vi "Dashboard Resize.vi"(6 "Cluster":T2={"Label Font Size"=24, "Data Font Size"=36, "String Font Size"=36}, 7 "Cluster 2":T1={"Label(%)"=0.4, "Data(%)"=0.4, "String(%)"=0.2}, 8 "error in (no error)":errorcluster, 9 "Cluster Size:Height":u32=134, 10 "Cluster Size:Width":u32=256, 11 "ClusterRef":refnum<vi>) -> (0 "error out":errorcluster, 1 "Bounds:Area Height":u32=134, 2 "Bounds:Area Width":u32=256)   [LabVIEW 2020, in "CSM-TagDashboard.lvlib"]
doc: "-- <b>Controls</b> --\n- <b>Cluster</b>:\n- <b>Cluster Size:Height</b>:\n- <b>Cluster Size:Width</b>:\n- <b>ClusterRef</b>:\n\n-- <b>Indicators</b> --\n- <b>Bounds:Area Height</b>:\n- <b>Bounds:Area Width</b>:"
uses:
  CSM-TagDashboard.lvlib
panel:
  out "引气压力P4 2":T3={"Label"="Label", "Value"="0.00", "String"="0.00"} caption="Digital"
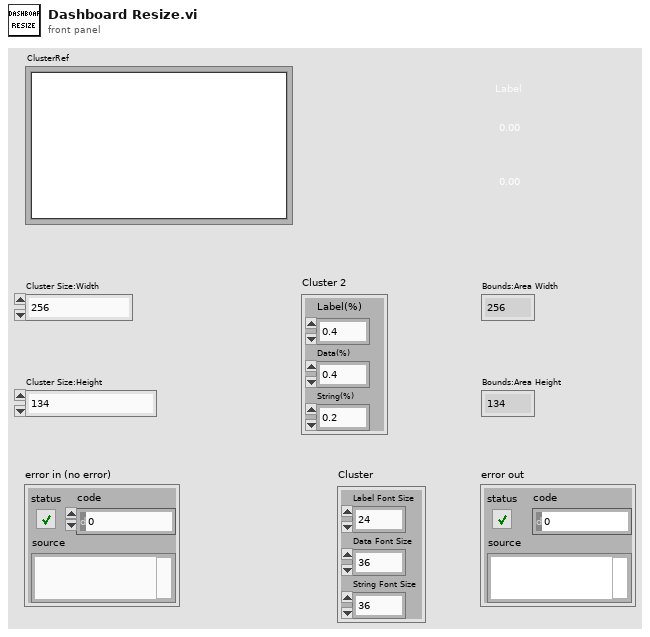
[diagram p1: front panel]
types:
  T1 = cluster{"Label(%)":dbl, "Data(%)":dbl, "String(%)":dbl}
  T2 = cluster{"Label Font Size":i32, "Data Font Size":i32, "String Font Size":i32}
  T3 = cluster{"Label":string, "Value":string, "String":string}
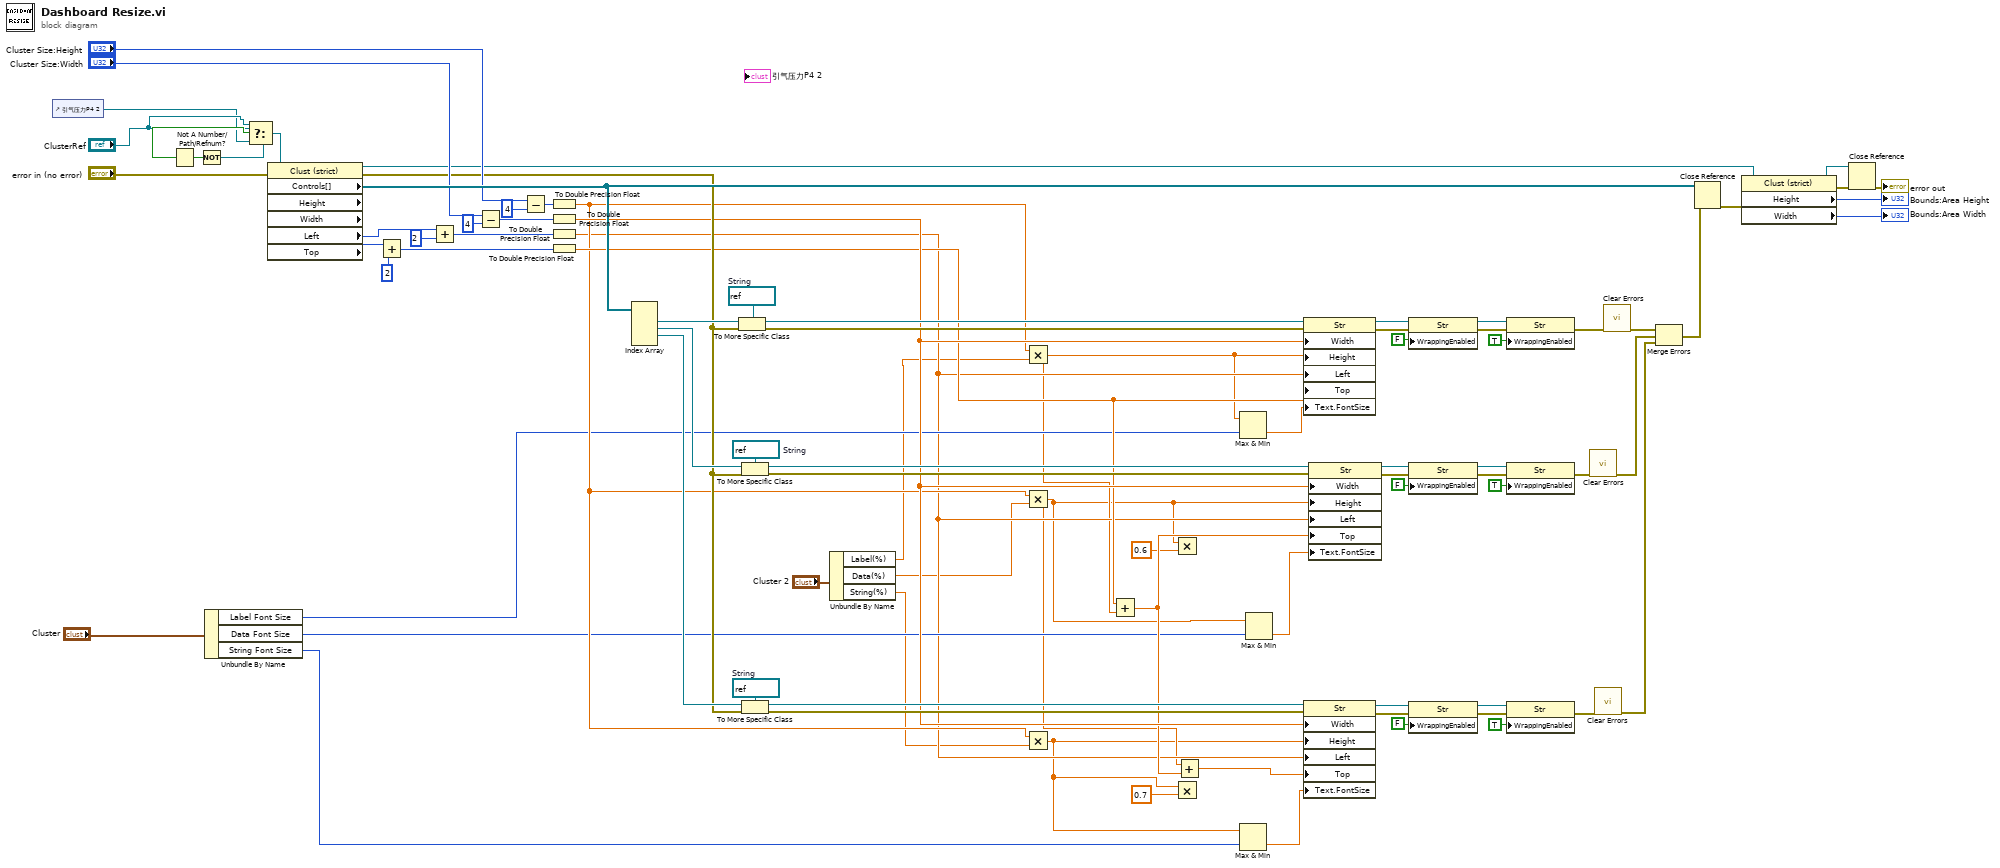
[diagram p0: block diagram]
diagram:
  w50 = refnum<vi> refnum  # String
  w81 = refnum<vi> refnum  # String
  w85 = refnum<vi> refnum  # String
  n1 = control-ref of="引气压力P4 2"() -> (w56:refnum<vi>)
  n2 = Not A Number/Path/Refnum?(number/path/refnum="ClusterRef") -> (NaN/Path/Refnum?=w15:bool)
  n3 = Not(x=w15) -> (.not. x?=w58:bool)
  n4 = Unbundle By Name("Cluster") -> ("Label Font Size"=w14:i32, "Data Font Size"=w13:i32, "String Font Size"=w12:i32)
  n5 = Select(t="ClusterRef", s=w58, f=w56) -> (s? t:f=w55:refnum<vi>)
  n6 = property on="Property Node" class="Clust (strict)" props=["Controls[]", "Height", "Width", "Left", "Top"](reference=w55, error in="error in (no error)") -> (reference out=w62:refnum<vi>, error out=w47:errorcluster, "Controls[]"=w86:refnum<vi>[], "Left"=w75:i32, "Top"=w72:i32)  [unwired: 2 out]
  n7 = Add(x=w72, y=2) -> (x+y=w53:i32)
  n8 = Add(x=w75, y=2) -> (x+y=w71:i32)
  n9 = Subtract(x="Cluster Size:Width", y=u32 4) -> (x-y=w78:u32)
  n10 = Subtract(x="Cluster Size:Height", y=u32 4) -> (x-y=w54:u32)
  n11 = To Double Precision Float(number=w54) -> (double precision float=w40:dbl)
  n12 = To Double Precision Float(number=w78) -> (double precision float=w46:dbl)
  n13 = To Double Precision Float(number=w71) -> (double precision float=w11:dbl)
  n14 = To Double Precision Float(number=w53) -> (double precision float=w42:dbl)
  n15 = Index Array(array=w86) -> (element #1=w83:refnum<vi>, element #2=w80:refnum<vi>, element #3=w48:refnum<vi>)  [unwired: 4 in, 1 out]
  n16 = To More Specific Class(target class=w85, reference=w83, error in=w47) -> (specific class reference=w84:refnum<vi>, error out=w68:errorcluster)
  n17 = To More Specific Class(target class=w81, reference=w80, error in=w47) -> (specific class reference=w82:refnum<vi>, error out=w69:errorcluster)
  n18 = To More Specific Class(target class=w50, reference=w48, error in=w47) -> (specific class reference=w49:refnum<vi>, error out=w51:errorcluster)
  n19 = Unbundle By Name("Cluster 2") -> ("Label(%)"=w7:dbl, "Data(%)"=w8:dbl, "String(%)"=w9:dbl)
  n20 = Multiply(x=w40, y=w7) -> (x*y=w3:dbl)
  n21 = Multiply(x=w40, y=w8) -> (x*y=w2:dbl)
  n22 = Multiply(x=w40, y=w9) -> (x*y=w1:dbl)
  n23 = Add(x=w42, y=w3) -> (x+y=w45:dbl)
  n24 = Multiply(x=w2, y=0.6) -> ()  [unwired: 1 out]
  n25 = Multiply(x=w1, y=0.7) -> ()  [unwired: 1 out]
  n26 = Add(x=w2, y=w45) -> (x+y=w52:dbl)
  n27 = Max & Min(x=w3, y=w14) -> (min(x,y)=w6:dbl)  [unwired: 1 out]
  n28 = Max & Min(x=w1, y=w12) -> (min(x,y)=w4:dbl)  [unwired: 1 out]
  n29 = Max & Min(x=w2, y=w13) -> (min(x,y)=w5:dbl)  [unwired: 1 out]
  n30 = property on="Property Node" class="Str"(reference=w84, error in=w68, "Width"=w46, "Height"=w3, "Left"=w11, "Top"=w42, "Text.FontSize"=w6) -> (reference out=w36:refnum<vi>, error out=w35:errorcluster)
  n31 = property on="Property Node" class="Str"(reference=w49, error in=w51, "Width"=w46, "Height"=w1, "Left"=w11, "Top"=w52, "Text.FontSize"=w4) -> (reference out=w18:refnum<vi>, error out=w17:errorcluster)
  n32 = property on="Property Node" class="Str"(reference=w82, error in=w69, "Width"=w46, "Height"=w2, "Left"=w11, "Top"=w45, "Text.FontSize"=w5) -> (reference out=w24:refnum<vi>, error out=w25:errorcluster)
  n33 = property on="Property Node" class="Str"(reference=w36, error in=w35, "WrappingEnabled"=FALSE ("Enable Wrapping")) -> (reference out=w31:refnum<vi>, error out=w32:errorcluster)
  n34 = property on="Property Node" class="Str"(reference=w24, error in=w25, "WrappingEnabled"=FALSE ("Enable Wrapping")) -> (reference out=w29:refnum<vi>, error out=w28:errorcluster)
  n35 = property on="Property Node" class="Str"(reference=w18, error in=w17, "WrappingEnabled"=FALSE ("Enable Wrapping")) -> (reference out=w19:refnum<vi>, error out=w20:errorcluster)
  n36 = property on="Property Node" class="Str"(reference=w31, error in=w32, "WrappingEnabled"=TRUE ("Enable Wrapping")) -> (error out=w30:errorcluster)  [unwired: 1 out]
  n37 = property on="Property Node" class="Str"(reference=w29, error in=w28, "WrappingEnabled"=TRUE ("Enable Wrapping")) -> (error out=w23:errorcluster)  [unwired: 1 out]
  n38 = property on="Property Node" class="Str"(reference=w19, error in=w20, "WrappingEnabled"=TRUE ("Enable Wrapping")) -> (error out=w16:errorcluster)  [unwired: 1 out]
  n39 = call <vilib>:"Clear Errors.vi"("error in (no error)"=w23) -> ("error out"=w38:errorcluster)  [unwired: 5 in, 1 out]
  n40 = call <vilib>:"Clear Errors.vi"("error in (no error)"=w16) -> ("error out"=w37:errorcluster)  [unwired: 5 in, 1 out]
  n41 = call <vilib>:"Clear Errors.vi"("error in (no error)"=w30) -> ("error out"=w39:errorcluster)  [unwired: 5 in, 1 out]
  n42 = Merge Errors(w39, w38, w37) -> (w79:errorcluster)
  n43 = Close Reference(reference=w86, error in (no error)=w79) -> (error out=w64:errorcluster)
  n44 = property on="Property Node" class="Clust (strict)"(reference=w62, error in=w64) -> (reference out=w61:refnum<vi>, error out=w63:errorcluster, "Height"=→"Bounds:Area Height":u32, "Width"=→"Bounds:Area Width":u32)
  n45 = Close Reference(reference=w61, error in (no error)=w63) -> (error out=→"error out":errorcluster)
